vi "pid_XY.vi"(6 "ready for output (T)":bool=TRUE, 8 "inputValid":bool=TRUE, 10 "fbParams":T2={"enable"=FALSE, "setPoint"=0.001007080078125, "pGain"=0.0, "iGain"=0.10000038146972656, "gainScale"=0}, 11 "input":fxp<+/-,24,16>) -> (0 "output valid":bool, 3 "output":T1, 4 "ready for input":bool)   [LabVIEW 2016]
uses:
  <vilib>/rvi/FXPMathLib/FxpInterpret/XNode/nifxpmath_Interpret.xnode
  <vilib>/rvi/FXPMathLib/FxpSub/XNode/nifxpmath_Sub.xnode
  <vilib>/rvi/FXPMathLib/FxpMul/XNode/nifxpmath_Multiplier.xnode
  <vilib>/rvi/FXPMathLib/FxpAdd/XNode/nifxpmath_Add.xnode
  <vilib>/rvi/FXPMathLib/sim/FxpSim.dll
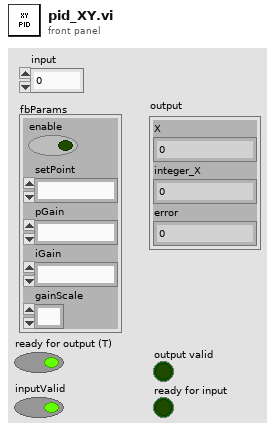
[diagram p1: front panel]
types:
  T1 = cluster{"X":fxp<+/-,28,1>, "integer_X":i16, "error":fxp<+/-,25,2>}
  T2 = cluster{"enable":bool, "setPoint":fxp<+/-,17,1>, "pGain":fxp<+/-,20,4>, "iGain":fxp<+/-,20,1>, "gainScale":i8}
  T3 = cluster{"X":fxp<+/-,28,1>, "X-integer":i16, "error":fxp<+/-,25,2>}
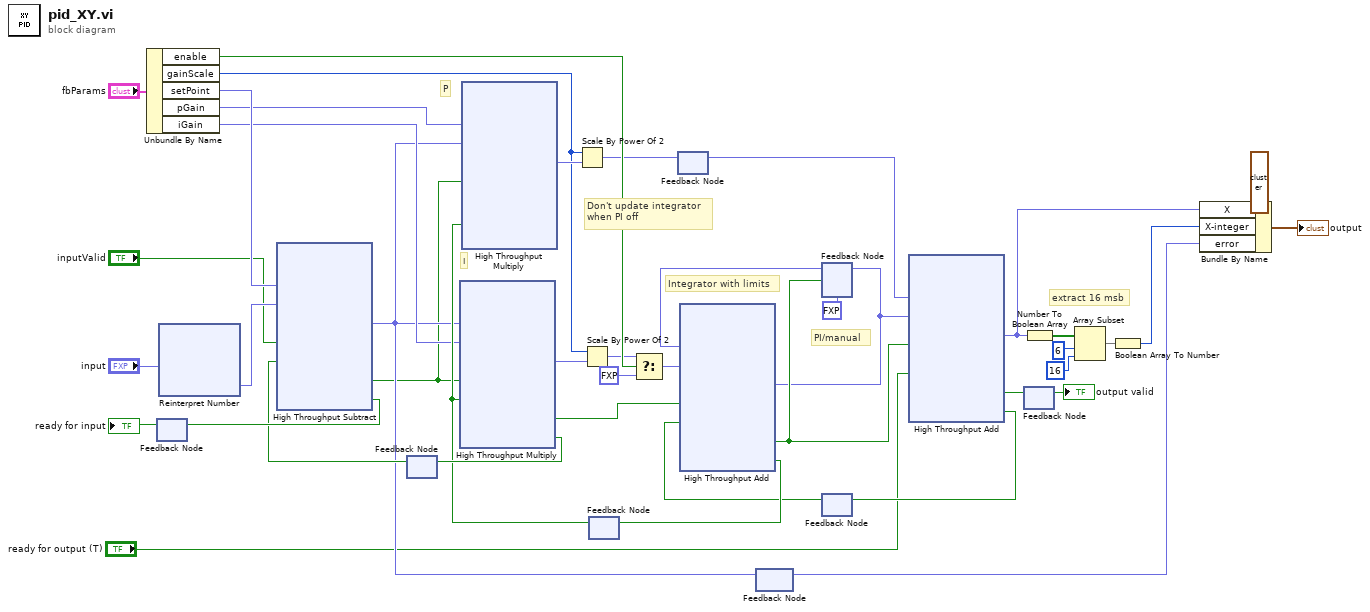
[diagram p0: block diagram]
diagram:
  # "Don't update integrator\nwhen PI off"
  # "PI/manual"
  # "I"
  # "P"
  # "Integrator with limits"
  # "extract 16 msb"
  n1 = Unbundle By Name("fbParams") -> ("enable"=w19:bool, "gainScale"=w23:i8, "setPoint"=w26:fxp<+/-,17,1>, "pGain"=w25:fxp<+/-,20,4>, "iGain"=w24:fxp<+/-,20,1>)
  n2 = feedback #1() -> (→"ready for input":bool)  [unwired: 1 in]
  n3 = xnode "Reinterpret Number"("x"="input") -> ("y"=w28:fxp<+/-,24,1>)
  n4 = feedback #2() -> (w40:bool)  [unwired: 1 in]
  n5 = xnode ("High Throughput Subtract")("x"=w26, "y"=w28, "input valid"="inputValid", "ready for output (T)"=w40) -> ("x-y"=w20:fxp<+/-,25,2>, "output valid"=w13:bool, "ready for input"=w43:bool)
  n6 = feedback-in #1(w43) -> ()
  n7 = feedback #3() -> (w37:bool)  [unwired: 1 in]
  n8 = xnode ("High Throughput Multiply")("x"=w20, "y"=w24, "input valid"=w13, "ready for output (T)"=w37) -> ("x*y"=w39:fxp<+/-,32,2>, "output valid"=w36:bool, "ready for input"=w41:bool)
  n9 = feedback-in #2(w41) -> ()
  n10 = xnode ("High Throughput Multiply")("x"=w25, "y"=w20, "input valid"=w13, "ready for output (T)"=w37) -> ("x*y"=w35:fxp<+/-,32,2>)  [unwired: 2 out]
  n11 = Scale By Power Of 2(n=w23, x=w35) -> (x*2^n=w5:fxp<+/-,32,2>)
  n12 = Scale By Power Of 2(n=w23, x=w39) -> (x*2^n=w8:fxp<+/-,32,2>)
  n13 = Select(t=w8, s=w19, f=fxp<+/-,32,2> 0.0) -> (s? t:f=w7:fxp<+/-,32,2>)
  n14 = feedback #4() -> (w33:fxp<+/-,32,2>)  [unwired: 1 in]
  n15 = feedback-in #4(w5) -> ()
  n16 = feedback #5() -> (w2:fxp<+/-,25,2>)  [unwired: 1 in]
  n17 = feedback-in #5(w20) -> ()
  n18 = feedback #6(fxp<+/-,32,4> -1.0 ("x+y")) -> (w9:fxp<+/-,32,4>)
  n19 = feedback #7() -> (w15:bool)  [unwired: 1 in]
  n20 = xnode ("High Throughput Add")("x"=w9, "y"=w7, "input valid"=w36, "ready for output (T)"=w15) -> ("x+y"=w1:fxp<+/-,32,4>, "output valid"=w4:bool, "ready for input"=w38:bool)
  n21 = feedback-in #3(w38) -> ()
  n22 = feedback-in #6(w1, w4) -> ()
  n23 = xnode ("High Throughput Add")("x"=w33, "y"=w1, "input valid"=w4, "ready for output (T)"="ready for output (T)") -> ("x+y"=w3:fxp<+/-,22,1>, "output valid"=w11:bool, "ready for input"=w34:bool)
  n24 = feedback-in #7(w34) -> ()
  n25 = feedback #8() -> (→"output valid":bool)  [unwired: 1 in]
  n26 = feedback-in #8(w11) -> ()
  n27 = Number To Boolean Array(number=w3) -> (Boolean array=w30:bool[])
  n28 = Array Subset(array=w30, index=6, length=16) -> (w29:bool[])
  n29 = Boolean Array To Number(Boolean array=w29) -> (number=w21:i16)
  n30 = Bundle By Name(cluster=T3 {"X"=0.0, "X-integer"=0, "error"=0.0} ("output"), "X"=w3, "X-integer"=w21, "error"=w2) -> (→"output":T3)
